vi "U3 4-Counter.vi"() -> ()   [LabVIEW 2021]
panel:
  in  "Case Constant\n(See Context Help)":bool=TRUE
  in  "Timer/Counter Pin Offset":u8
  in  "Reset Counters":bool
  in  "Iteration Inverval (milliseconds)":u32=100
  in  "# of firmware counters to enable":u32=2
  out "Counter1":u32
  out "Counter0":u32
  out "Timer Value Reads":u32[](array[numeric])
  out "Iteration":i32
  in  "error in":errorcluster
  in  "Address":string="1"
  in  "FirstFound":bool=TRUE
  in  "stop":bool
  out "error out":errorcluster
  out "Error Message":string
  # "Enables 0-2 firmware counters (timers) and both hardware counters, then reads\nall at the specified interval.  Timers will be assigned to pins starting with FIO0 plus\npin offset, and the hardware counters will get the next two pins after all timers."
  # "Firmware Counter 0"
  # "Firmware Counter 1"
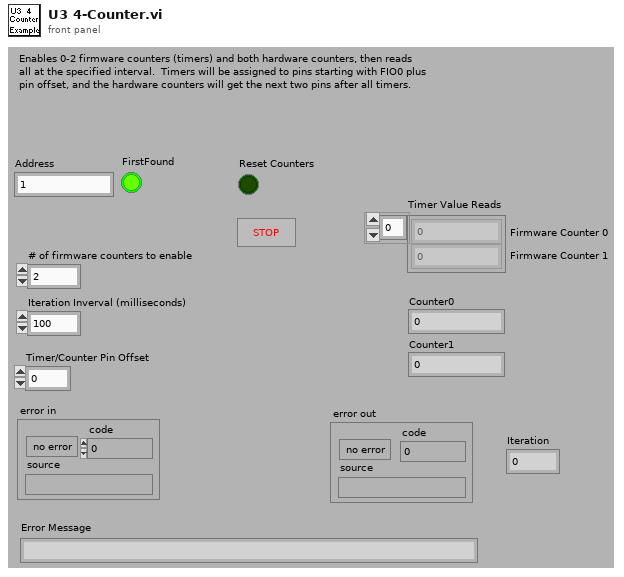
[diagram p1: front panel]
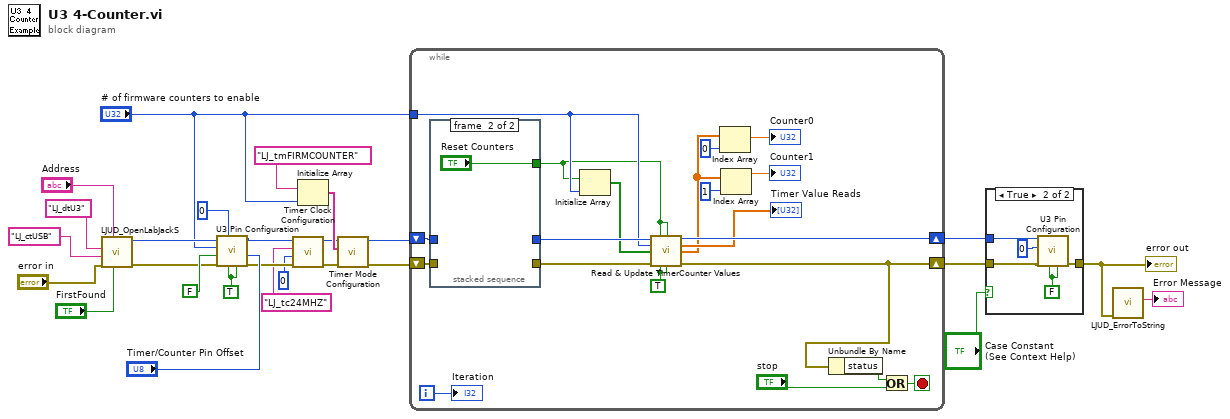
[diagram p0: block diagram]
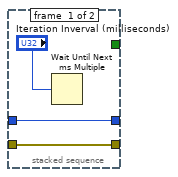
[diagram p3: hidden frame]
diagram:
  w17 = TRUE ("Enable Counter0")
  n1 = call "LJUD_OpenLabJackS.vi"("FirstFound"="FirstFound", "Address"="Address", "error in"="error in", "ConnectionType"="LJ_ctUSB", "DeviceType"="LJ_dtU3") -> ("error out"=w10:errorcluster, "Handle"=w12:i32)  [unwired: 4 in, 1 out]
  n2 = call "U3 Pin Configuration.vi"("Timer/Counter Pin Offset"="Timer/Counter Pin Offset", "Enable Counter1"=w17, "Enable Counter0"=w17, "FIO/EIO Analog Enable"=u8 0 ("FIO Analog Enable"), "error in"=w10, "Enable DAC1"=FALSE, "Number of Timers Enabled"="# of firmware counters to enable", "Handle In"=w12) -> ("error out"=w4:errorcluster, "Handle Out"=w3:i32)  [unwired: 2 in]
  n3 = call "Timer Clock Configuration.vi"("error in"=w4, "Timer Clock Divisor"=0, "Timer Clock Base"="LJ_tc24MHZ", "Handle In"=w3) -> ("error out"=w5:errorcluster, "Handle Out"=w6:i32)  [unwired: 6 in]
  n4 = Initialize Array("LJ_tmFIRMCOUNTER", "# of firmware counters to enable") -> (w15:string[])
  n5 = call "Timer Mode Configuration.vi"("error in"=w5, "TimerModes"=w15, "Handle In"=w6) -> ("error out"=w9:errorcluster, "Handle Out"=w11:i32)  [unwired: 7 in]
  n6 = while {
    shift-right: [w39] -> w23
    shift-left: w11 -> [w47]
    shift-right: [w38] -> w24
    shift-left: w9 -> [w46]
    tunnel: "# of firmware counters to enable" -> [w37]
    i -> [w40]
    stop <- w43 stop-if-true
    w28 = TRUE ("Reset Counter0")
    n7 = stacked-sequence {
      tunnel: [w50 _] -> w45
      tunnel: [w49 _] -> w44
      tunnel: w47 -> [w50 _]
      tunnel: w46 -> [w49 _]
      tunnel: [_ "Reset Counters"] -> w32
      frame #0 {
        n8 = Wait Until Next ms Multiple(millisecond multiple="Iteration Inverval (milliseconds)") -> ()  [unwired: 1 out]
      }
      frame #1 {
      }
    }
    n9 = Initialize Array(w32, w37) -> (w36:bool[])
    n10 = call "Read & Update TimerCounter Values.vi"("Handle In"=w45, "Reset Counter0"=w32, "Reset Counter1"=w32, "# Timers to Read"=w37, "UpdateReset Timers"=w36, "error in"=w44, "Read Counter0"=w28, "Read Counter1"=w28) -> ("Handle Out"=w39:i32, "Timer Value Reads"=→"Timer Value Reads":dbl[], "Counter Value Reads"=w30:dbl[], "error out"=w38:errorcluster)  [unwired: 4 in]
    n11 = Index Array(array=w30, index=0 ("Index")) -> (element=→"Counter0":dbl)
    n12 = Index Array(array=w30, index=1 ("Index")) -> (element=→"Counter1":dbl)
    n13 = Unbundle By Name(w38) -> ("status"=w42:bool)
    n14 = Or(x=w42, y="stop") -> (x .or. y?=w43:bool)
    "Iteration" <- w40
  }
  n15 = case shown="True" "Case Constant\n(See Context Help)" {
    tunnel: w24 -> [w52 w57]
    tunnel: w23 -> [_ w56]
    tunnel: [w52 w55] -> w26
    frame False {
    }
    frame True {
      w54 = FALSE ("Enable Counter0")
      n16 = call "U3 Pin Configuration.vi"("Enable Counter1"=w54, "Enable Counter0"=w54, "error in"=w57, "Number of Timers Enabled"=u16 0, "Handle In"=w56) -> ("error out"=w55:errorcluster)  [unwired: 5 in, 1 out]
    }
  }
  "error out" <- w26
  n17 = call "LJUD_ErrorToString.vi"("error in"=w26) -> ("String"=→"Error Message":string)  [unwired: 10 in]
